vi "Z_CBF_F.vi"(8 "平移采样点信息":dbl[][](array[numeric]), 9 "禁用的索引 (列)":i32, 11 "Waveform":waveform(dbl)[](array[waveform])) -> (3 "数组输出":dbl[][](array[numeric]))   [LabVIEW 2018]
uses:
  <vilib>/measure/maspectr.llb/FFT Spectrum (Real-Im) for 1 Chan.vi
  <vilib>/Analysis/Matrix/Numeric/Conversions/Array To Matrix - CA.vi
  <vilib>/Analysis/Matrix/Numeric/Multiply/Multiply - CM,CM.vi
  <vilib>/Analysis/Matrix/Numeric/Conversions/Matrix To Array - CM.vi
  <vilib>/Analysis/Matrix/NI_Matrix.lvlib
  <vilib>/measure/NI_MAPro.lvlib
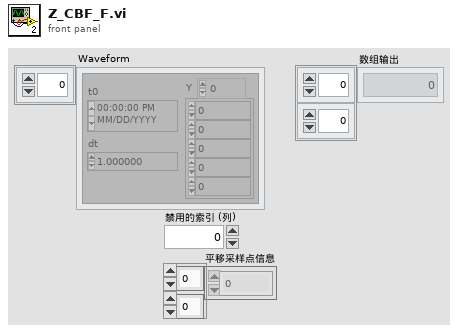
[diagram p1: front panel]
types:
  T1 = cluster{"f0":dbl, "df":dbl, "imaginary part":dbl[]}
  T2 = typedef "NI_Matrix.lvlib/ComplexMatrix.ctl" = cdb[][]
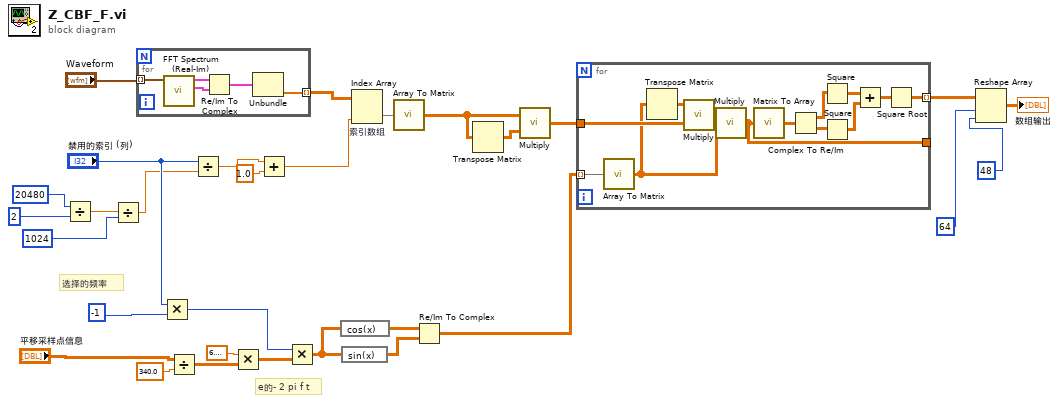
[diagram p0: block diagram]
diagram:
  # "选择的频率"
  # "e的- 2 pi f t"
  n1 = Divide(x=20480, y=2) -> (x/y=w4:dbl)
  n2 = Divide(x=w4, y=1024) -> (x/y=w3:dbl)
  n3 = for {
    tunnel: "Waveform" -> [w31] mode=indexing
    tunnel: [w35] -> w30 mode=indexing
    n4 = call-poly <vilib>:"FFT Spectrum (Real-Im).vi"("time signal"=w31) -> ("imaginary part"=w33:T1, "real part"=w34:cluster{"f0":dbl, "df":dbl, "real part":dbl[]})  [unwired: 6 in, 3 out]
    n5 = Re/Im To Complex(1:w33, 2:w34) -> (0:w32:cluster{"f0":cdb, "df":cdb, cdb[]})
    n6 = Unbundle(w32) -> (w35:cdb[])  [unwired: 2 out]
  }
  n7 = Multiply(x="禁用的索引 (列)", y=-1) -> (x*y=w19:i32)
  n8 = Divide(x="平移采样点信息", y=340.0) -> (x/y=w18:dbl[][])
  n9 = Divide(x="禁用的索引 (列)", y=w3) -> (x/y=w2:dbl)
  n10 = Multiply(x=6.283185307179586, y=w18) -> (x*y=w15:dbl[][])
  n11 = Add(x=w2, y=1.0) -> (x+y=w20:dbl)
  n12 = Multiply(x=w19, y=w15) -> (x*y=w10:dbl[][])
  n13 = expression code="cos(x)"(w10) -> (w16:dbl[][])
  n14 = expression code="sin(x)"(w10) -> (w17:dbl[][])
  n15 = Index Array "索引数组"(array=w30, index (col)=w20) -> (element=w22:cdb[])  [unwired: 1 in]
  n16 = call-poly <vilib>:"Array To Matrix.vi"("Complex 1D Array"=w22) -> ("Complex Matrix (Column Vector)"=w25:T2)
  n17 = Re/Im To Complex(1:w17, 2:w16) -> (0:w9:cdb[][])
  n18 = Transpose Matrix(1:w25) -> (0:w24:T2)
  n19 = call-poly <vilib>:"Multiply.vi"("Complex Matrix B"=w24, "Complex Matrix A"=w25) -> ("A * B"=w23:T2)
  n20 = for {
    tunnel: w9 -> [w48] mode=indexing
    tunnel: w23 -> [w46]
    tunnel: [w38] -> _
    tunnel: [w36] -> w26 mode=indexing
    n21 = call-poly <vilib>:"Array To Matrix.vi"("Complex 1D Array"=w48) -> ("Complex Matrix (Column Vector)"=w44:T2)
    n22 = Transpose Matrix(1:w44) -> (0:w47:T2)
    n23 = call-poly <vilib>:"Multiply.vi"("Complex Matrix B"=w46, "Complex Matrix A"=w47) -> ("A * B"=w45:T2)
    n24 = call-poly <vilib>:"Multiply.vi"("Complex Matrix B"=w44, "Complex Matrix A"=w45) -> ("A * B"=w38:T2)
    n25 = call-poly <vilib>:"Matrix To Array.vi"("Complex Matrix"=w38) -> ("Complex 2D Array"=w37:cdb[][])
    n26 = Complex To Re/Im ("Complex To Cartesian.vi")(x + iy=w37) -> (x=w43:dbl[][], y=w42:dbl[][])
    n27 = Square(x=w43) -> (x^2=w40:dbl[][])
    n28 = Square(x=w42) -> (x^2=w39:dbl[][])
    n29 = Add ("Add.vi")(x=w40, y=w39) -> (x+y=w41:dbl[][])
    n30 = Square Root ("Square Root.vi")(x=w41) -> (sqrt(x)=w36:dbl[][])
  }
  n31 = Reshape Array(w26, 64 ("维数大小"), 48 ("维数大小")) -> (→"数组输出":dbl[][])
